vi "Turn To Angle Teleop.vi"(8 "Z Axis":dbl, 10 "POV":i16) -> (2 "Adjustment Voltage":dbl)   [LabVIEW 2017]
uses:
  <vilib>/Rock Robotics/Network Tables/NT Read Number.vi
  <vilib>/addons/control/pid/pid.llb/PID (DBL).vi
  <vilib>/addons/control/pid/NI_PID_pid.lvlib
panel:
  # ".0202"
  # "0"
  # ".0032150"
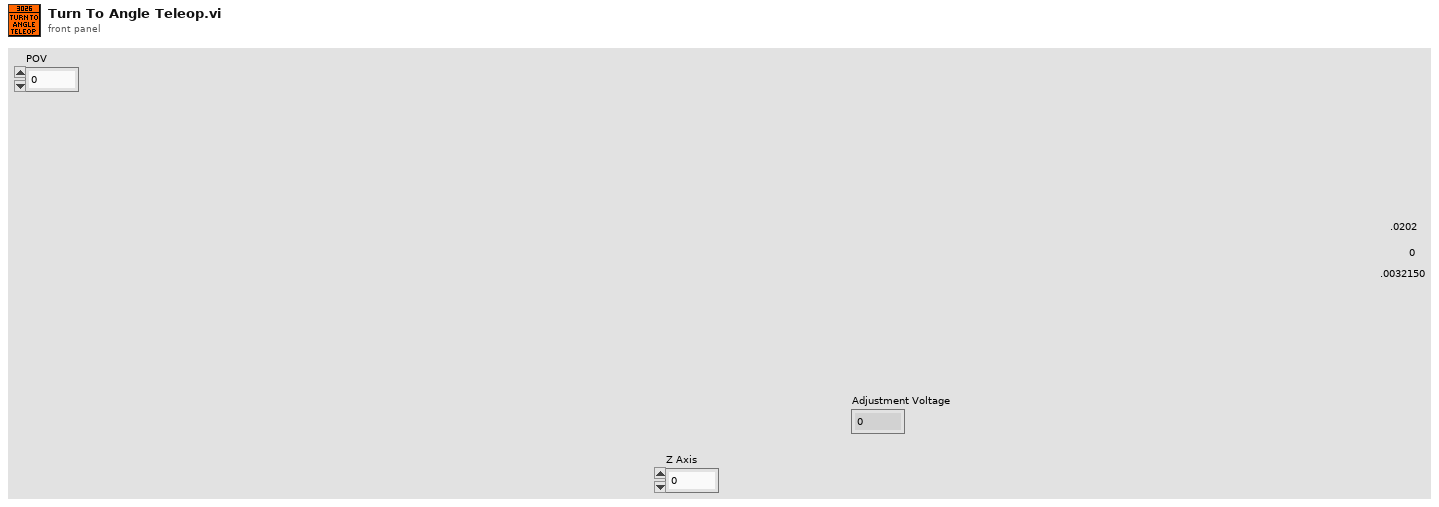
[diagram p1: front panel]
types:
  T1 = cluster{"proportional gain (Kc)":dbl, "integral time (Ti, min)":dbl, "derivative time (Td, min)":dbl}
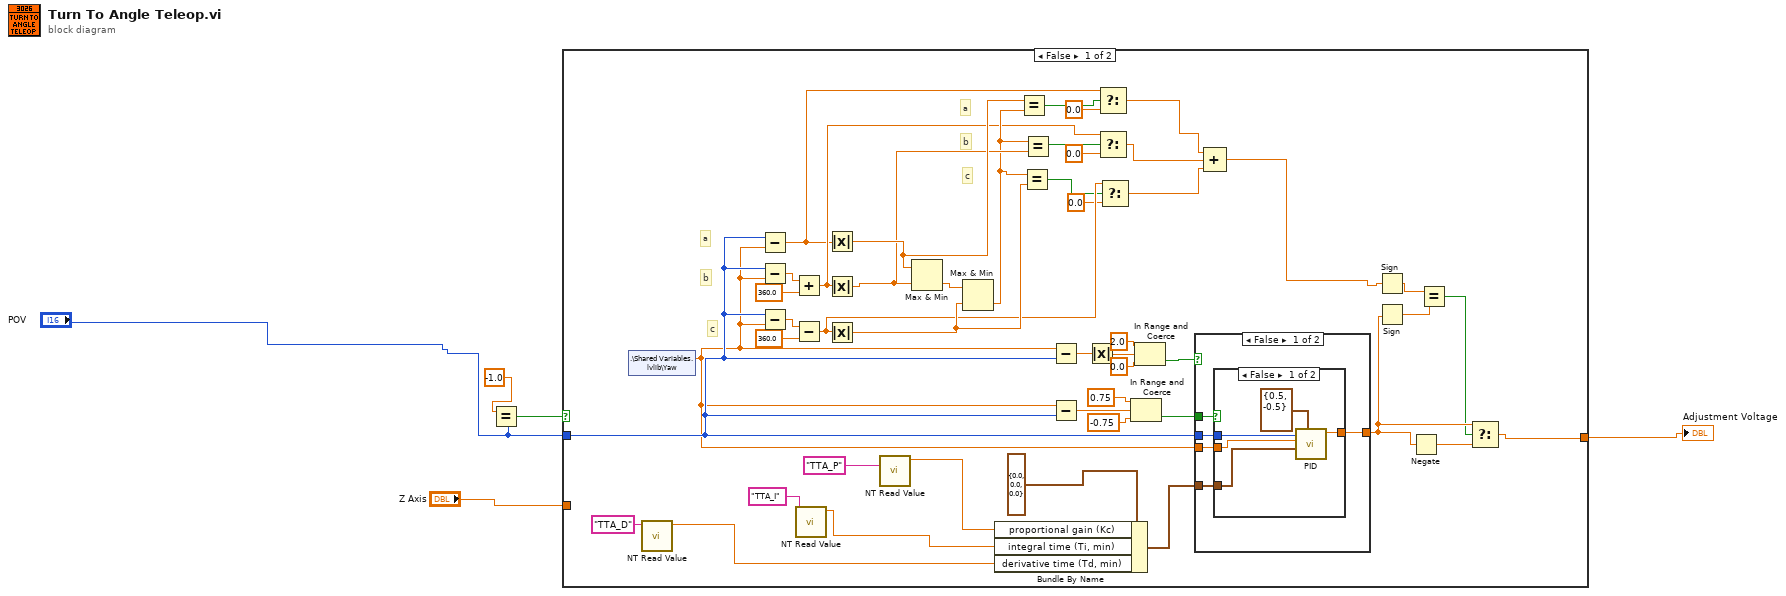
[diagram p0: block diagram]
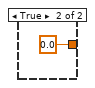
[diagram p2: hidden frame]
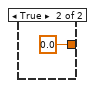
[diagram p3: hidden frame]
diagram:
  n1 = Equal?(x=-1.0, y="POV") -> (x = y?=w1:bool)
  n2 = case shown="False" w1 {
    tunnel: "POV" -> [w39 _]
    tunnel: [w19 w65] -> w4
    tunnel: "Z Axis" -> [_ w65]
    frame False {
      # "c"
      # "b"
      # "a"
      # "c"
      # "b"
      # "a"
      n3 = shared-variable ".\\Shared Variables.lvlib\\Yaw"() -> (w38:dbl)  [unwired: 1 in, 1 out]
      n4 = call-poly <vilib>:"NT Read Value.vi"("Name"="TTA_D") -> ("Numeric"=w9:dbl)  [unwired: 9 in, 1 out]
      n5 = Subtract(x=w39, y=w38) -> (x-y=w30:dbl)
      n6 = Subtract(x=w39, y=w38) -> (x-y=w43:dbl)
      n7 = Subtract(x=w39, y=w38) -> (x-y=w41:dbl)
      n8 = Add(x=w43, y=360.0) -> (x+y=w31:dbl)
      n9 = Subtract(x=w41, y=360.0) -> (x-y=w29:dbl)
      n10 = call-poly <vilib>:"NT Read Value.vi"("Name"="TTA_I") -> ("Numeric"=w10:dbl)  [unwired: 9 in, 1 out]
      n11 = Absolute Value(x=w30) -> (abs(x)=w36:dbl)
      n12 = Absolute Value(x=w31) -> (abs(x)=w35:dbl)
      n13 = Absolute Value(x=w29) -> (abs(x)=w33:dbl)
      n14 = call-poly <vilib>:"NT Read Value.vi"("Name"="TTA_P") -> ("Numeric"=w11:dbl)  [unwired: 9 in, 1 out]
      n15 = Max & Min(x=w36, y=w35) -> (min(x,y)=w37:dbl)  [unwired: 1 out]
      n16 = Max & Min(x=w37, y=w33) -> (min(x,y)=w34:dbl)  [unwired: 1 out]
      n17 = Bundle By Name(cluster=T1 {"proportional gain (Kc)"=0.0, "integral time (Ti, min)"=0.0, "derivative time (Td, min)"=0.0} ("PID gains"), "proportional gain (Kc)"=w11, "integral time (Ti, min)"=w10, "derivative time (Td, min)"=w9) -> (w13:T1)
      n18 = Equal?(x=w36, y=w34) -> (x = y?=w28:bool)
      n19 = Equal?(x=w34, y=w33) -> (x = y?=w27:bool)
      n20 = Equal?(x=w34, y=w35) -> (x = y?=w32:bool)
      n21 = Subtract(x=w38, y=w39) -> (x-y=w50:dbl)
      n22 = Subtract(x=w38, y=w39) -> (x-y=w48:dbl)
      n23 = Absolute Value(x=w50) -> (abs(x)=w49:dbl)
      n24 = Select(t=w30, s=w28, f=0.0) -> (s? t:f=w23:dbl)
      n25 = Select(t=w31, s=w32, f=0.0) -> (s? t:f=w22:dbl)
      n26 = Select(t=w29, s=w27, f=0.0) -> (s? t:f=w21:dbl)
      n27 = In Range and Coerce(upper limit=0.75, x=w48, lower limit=-0.75) -> (In Range?=w45:bool)  [unwired: 1 out]
      n28 = In Range and Coerce(upper limit=2.0, x=w49, lower limit=0.0) -> (In Range?=w44:bool)  [unwired: 1 out]
      n29 = case shown="False" w44 {
        tunnel: w38 -> [w57 _]
        tunnel: w45 -> [w54 _]
        tunnel: w39 -> [w56 _]
        tunnel: [w55 0.0 ("output")] -> w17
        tunnel: w13 -> [w53 _]
        frame False {
          n30 = case shown="False" w54 {
            tunnel: w57 -> [w62 _]
            tunnel: w56 -> [w59 _]
            tunnel: [w60 0.0 ("output")] -> w55
            tunnel: w53 -> [w58 _]
            frame False {
              n31 = call-poly <vilib>:"PID.vi"("output range"=cluster{"output high":dbl, "output low":dbl} {"output high"=0.5, "output low"=-0.5}, "PID gains"=w58, "process variable"=w62, "setpoint"=w59) -> ("output"=w60:dbl)  [unwired: 6 in, 1 out]
            }
            frame True {
            }
          }
        }
        frame True {
        }
      }
      n32 = Compound Arithmetic op=ADD(w23, w22, w21) -> (w18:dbl)
      n33 = Sign(1:w18) -> (0:w16:dbl)
      n34 = Sign(1:w17) -> (0:w14:dbl)
      n35 = Negate(x=w17) -> (-x=w20:dbl)
      n36 = Equal?(x=w16, y=w14) -> (x = y?=w15:bool)
      n37 = Select(t=w17, s=w15, f=w20) -> (s? t:f=w19:dbl)
    }
    frame True {
    }
  }
  "Adjustment Voltage" <- w4
